vi "WIZARD.vi"() -> ()   [LabVIEW 2015]
uses:
  Controls/FGV_Options.ctl
  Controls/HID State.ctl
panel:
  out "String":string="System architecture (Windows Host and FPGA); LED Matrix (combination of 32x32 matrices in 2 rows and 3 columns); diving a little: row addressing are made in pair of n, n+15 rows. E.g., address 0 corresponds to rows 0 and 16 and ADRESS \"0xF\" or \"15\" corresponds to rows 15 and 31."
  in  "Button Back":bool
  out "2D Picture":picture
  out "Step Title":string
  out "Active Steps":string[](array[string])=["", "", "2. Coletando Dados Da Câmera!", "", "", "", ""]
  out "Steps Background":string[](array[string])=["Quer aprender como funciona a Demo?", "1. Vamos Começar", "2. Coletando Dados Da Câmera!", "3. Transformando em Vetor", "4. Enviando para o FPGA", "5. Colocando nas Memórias", "6. Gerando"]
  in  "Button Cancel":bool
  in  "Button Next":bool
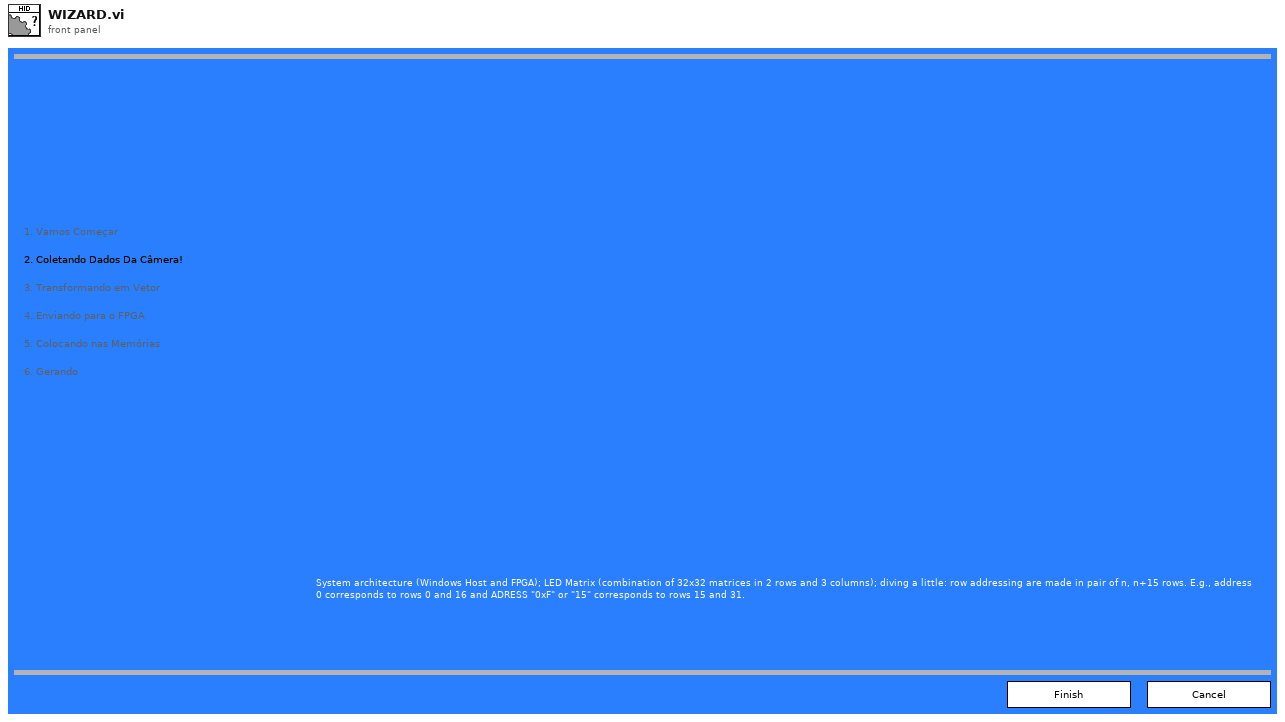
[diagram p1: front panel]
types:
  T1 = typedef "FGV_Options.ctl" = enum16{"Read from File", "Write to File", "Get", "Set"}
  T2 = cluster{"Steps":string[], "Images":picture[], "Step Counter":i32}
  T3 = typedef "HID Data.ctl" = cluster{"IMAQdx Session":T4, "Resampled Image":T5, "Low Level Grab":T5, "X Resolution":i32, "Y Resolution":i32, "Image Threshold":u8, "Reset Value":i32, "FIFO Timer":u16, "Row Timer":u32, "Memory Writer Timer":u8, "Color":enum16{"Green", "Blue", "Red", "White", "Pink", "Yellow", "Turquoise", "Black"}, "Top":bool[][], "Bottom":bool[][], "Timeout (ms)":i32, "Menu Tag":string, "Color Background":enum16{"Green", "Blue", "Red", "White", "Pink", "Yellow", "Turquoise", "Black"}, "FPGA VI Reference":refnum<k20>, "Next Steps":T6[], "Turn off LED Matrix":bool, "FPGA Alias":string, "FPGA Bitfile":path, "Localized Texts":cluster{"Status Text":cluster{"Status Text Table":string[], "Status Text Index":i32}, "Controls":cluster{"Control Text Table":string[], "Control Text Index":i32}, "Titles":cluster{"Titles Text Table":string[], "Titles Text Index":i32}}, "Language":u16}
  T4 = typedef "IMAQdx.ctl" = refnum<k21>
  T5 = typedef "IMAQ Image.ctl" = refnum<image>
  T6 = typedef "HID State.ctl" = enum16{"Initialize", "Set FPGA Parametes", "Set Camera Parameters", "Set LED Matrix Parameters", "Initialize FPGA Interface", "Initialize Camera", "Start FPGA VI", "Start Camera", "Wait for Event", "Update UI", "Acquire", "Process Image", "Get Boolean Arrays", "Send to FPGA", "Menu Pop-Up", "Menu Actions", "Handle Errors", "Close Camera", "Close FPGA", "Stop", "Exit"}
  T7 = enum8{"Enabled", "Disabled", "Disabled and Grayed Out"}
  T8 = typedef "imagedata.ctl" = cluster{"image type":i32, "image depth":i32, "image":u8[], "mask":u8[], "colors":u32[], "Rectangle":cluster{"left":i16, "top":i16, "right":i16, "bottom":i16}}
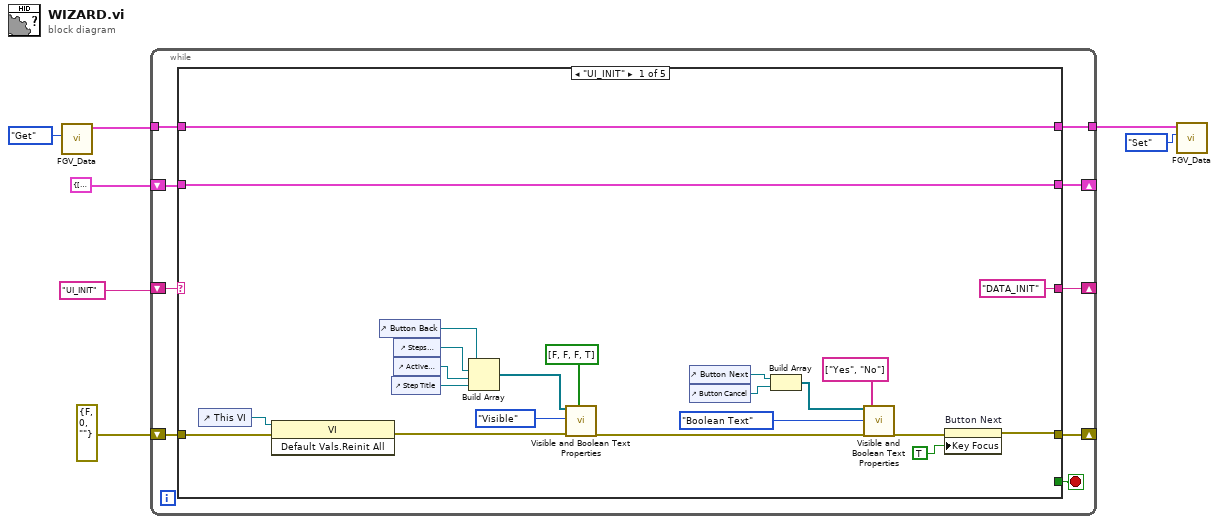
[diagram p0: block diagram]
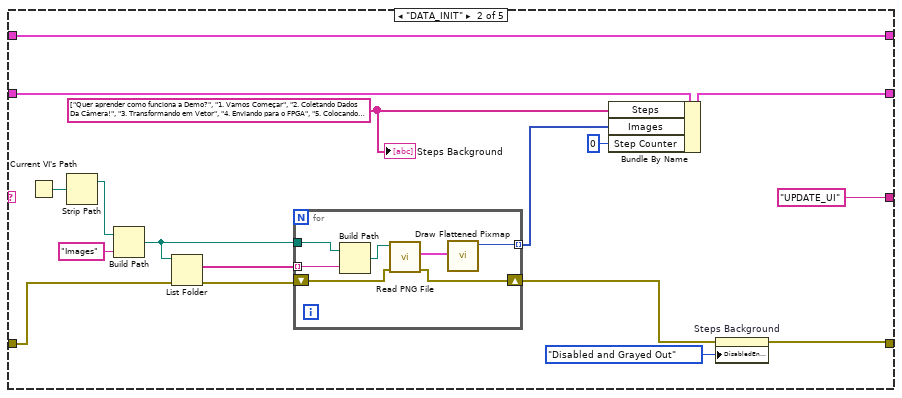
[diagram p2: hidden frame]
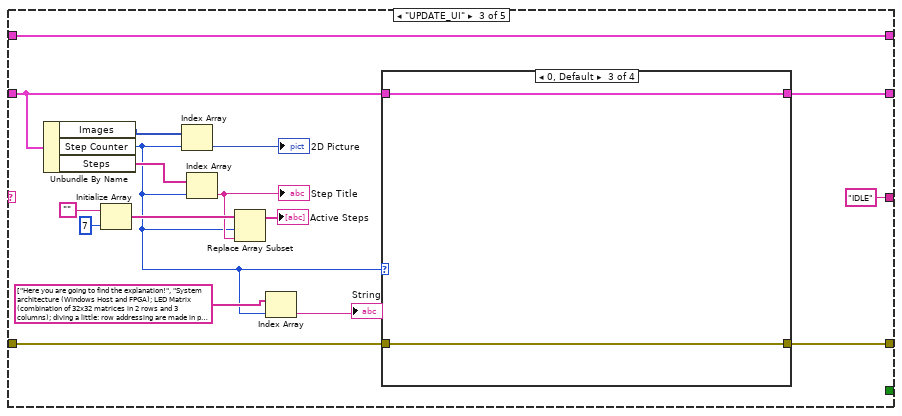
[diagram p3: hidden frame]
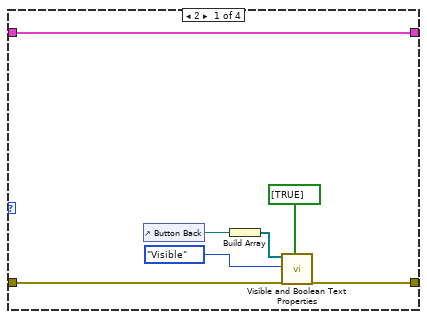
[diagram p4: hidden frame]
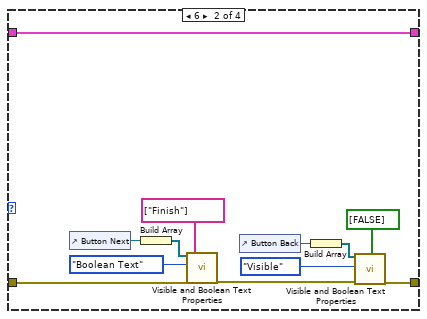
[diagram p5: hidden frame]
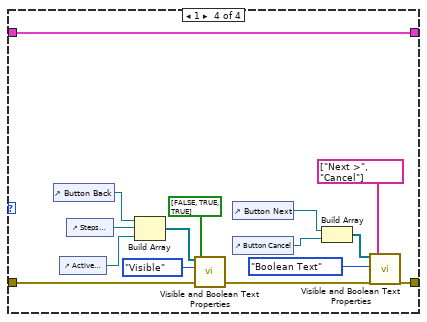
[diagram p6: hidden frame]
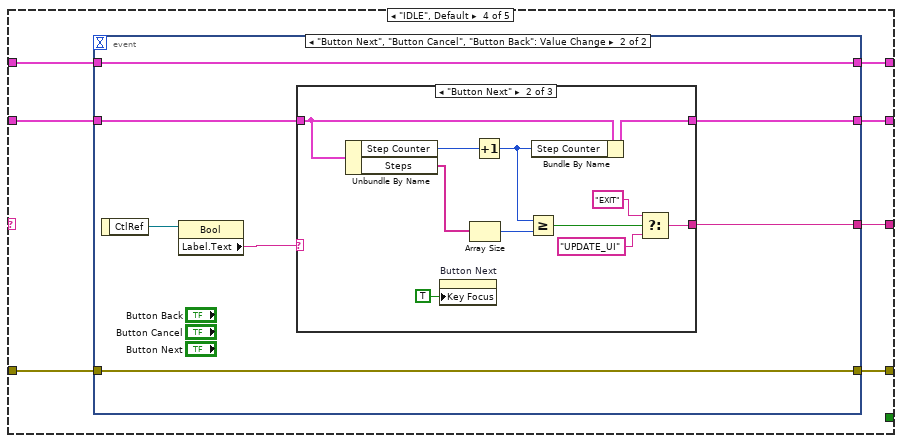
[diagram p7: hidden frame]
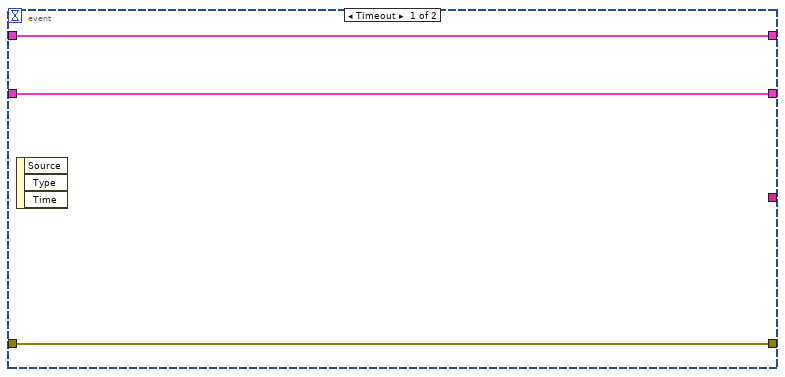
[diagram p8: hidden frame]
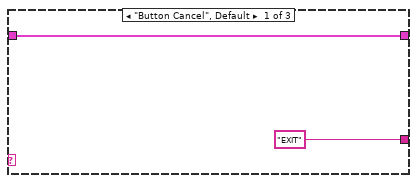
[diagram p9: hidden frame]
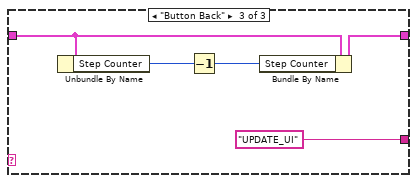
[diagram p10: hidden frame]
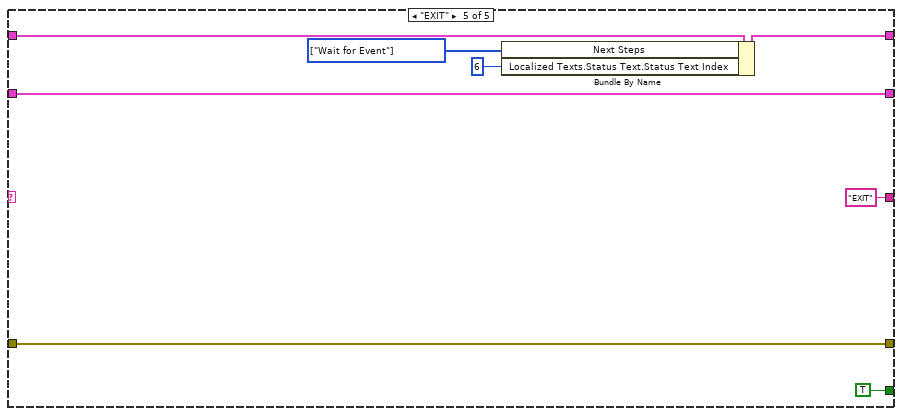
[diagram p11: hidden frame]
diagram:
  n1 = call "FGV_Data.vi"("Option"=FGV_Options."Get") -> ("Data Out"=w4:T3)  [unwired: 9 in, 1 out]
  n2 = while {
    shift-right: [w14] -> _
    shift-left: T2 {"Steps"=[], "Images"=[], "Step Counter"=0} -> [w15]
    shift-right: [w13] -> _
    shift-left: "UI_INIT" -> [w16]
    shift-right: [w11] -> _
    shift-left: errorcluster {"status"=FALSE, "code"=0, "source"=""} ("error constant") -> [w10]
    tunnel: w4 -> [w9]
    tunnel: [w8] -> w2
    stop <- w12 stop-if-true
    n3 = case shown="\"UI_INIT\"" w16 {
      tunnel: w15 -> [w38 w55 w71 w122 w158]
      tunnel: [w38 w53 w70 w121 w158] -> w14
      tunnel: ["DATA_INIT" "UPDATE_UI" "IDLE" w120 "EXIT"] -> w13
      tunnel: [_ _ _ _ TRUE] -> w12
      tunnel: [w19 w41 w68 w118 w155] -> w11
      tunnel: w10 -> [w18 w44 w69 w119 w155]
      tunnel: w9 -> [w17 w40 w66 w117 w154]
      tunnel: [w17 w40 w66 w116 w153] -> w8
      frame "UI_INIT" {
        n4 = control-ref of="This VI"() -> (w37:refnum<vi>)
        n5 = invoke class="VI" method="Default Vals.Reinit All"(reference=w37, error in=w18) -> (error out=w23:errorcluster)  [unwired: 1 in, 2 out]
        n6 = control-ref of="Button Back"() -> (w29:refnum<vi>)
        n7 = control-ref of="Step Title"() -> (w24:refnum<vi>)
        n8 = control-ref of="Steps Background"() -> (w25:refnum<vi>)
        n9 = control-ref of="Active Steps"() -> (w26:refnum<vi>)
        n10 = Build Array(w29, w25, w26, w24) -> (w27:refnum<vi>[])
        n11 = call "Visible and Boolean Text Properties.vi"("Control References"=w27, "Option"=enum16{"Visible", "Boolean Text"}."Visible", "error in (no error)"=w23, "Controls Visible Property Values"=bool[] [FALSE, FALSE, FALSE, TRUE]) -> ("error out"=w21:errorcluster)  [unwired: 15 in]
        n12 = control-ref of="Button Next"() -> (w31:refnum<vi>)
        n13 = control-ref of="Button Cancel"() -> (w32:refnum<vi>)
        n14 = Build Array(w31, w32) -> (w33:refnum<vi>[])
        n15 = call "Visible and Boolean Text Properties.vi"("Control References"=w33, "Option"=enum16{"Visible", "Boolean Text"}."Boolean Text", "error in (no error)"=w21, "Boolean Text Array"=string[] ["Yes", "No"]) -> ("error out"=w20:errorcluster)  [unwired: 15 in]
        n16 = property on="Button Next" class="Bool"(error in=w20, "Key Focus"=TRUE) -> (error out=w19:errorcluster)  [unwired: 1 in, 1 out]
      }
      frame "DATA_INIT" {
        w47 = string[] ["Quer aprender como funciona a Demo?", "1. Vamos Começar", "2. Coletando Dados Da Câmera!", "3. Transformando em Vetor", "4. Enviando para o FPGA", "5. Colocando nas Memórias", "6. Gerando"]
        n17 = Current VI's Path() -> (path=w52:path)
        n18 = Strip Path(path=w52) -> (stripped path=w39:path)  [unwired: 1 out]
        n19 = Build Path(base path=w39, name or relative path="Images") -> (appended path=w50:path)
        n20 = List Folder(path=w50, error in=w44) -> (filenames=w54:string[], error out=w43:errorcluster)  [unwired: 2 in, 2 out]
        n21 = for {
          tunnel: w54 -> [w62] mode=indexing
          tunnel: w50 -> [w61]
          tunnel: [w58] -> w49 mode=indexing
          shift-right: [w56] -> w42
          shift-left: w43 -> [w57]
          n22 = Build Path(base path=w61, name or relative path=w62) -> (appended path=w60:path)
          n23 = call <vilib>:"Read PNG File.vi"("error in (no error)"=w57, "path to PNG file"=w60) -> ("error out"=w56:errorcluster, "image data"=w59:T8)  [unwired: 7 in, 1 out]
          n24 = call <vilib>:"Draw Flattened Pixmap.vi"("image data"=w59) -> ("new picture"=w58:picture)  [unwired: 8 in]
        }
        n25 = Bundle By Name(cluster=w55, "Steps"=w47, "Images"=w49, "Step Counter"=0) -> (w53:T2)
        n26 = property on="Steps Background" class="Arr (strict)"(error in=w42, "DisabledEnum"=T7."Disabled and Grayed Out" ("Disabled")) -> (error out=w41:errorcluster)  [unwired: 1 in, 1 out]
        "Steps Background" <- w47
      }
      frame "UPDATE_UI" {
        n27 = Unbundle By Name(w71) -> ("Images"=w77:picture[], "Step Counter"=w63:i32, "Steps"=w67:string[])
        n28 = Initialize Array("", 7 ("dimension size")) -> (w75:string[])
        n29 = Index Array(array=w77, index=w63) -> (element=→"2D Picture":picture)
        n30 = Index Array(array=w67, index=w63) -> (element=w73:string)
        "Step Title" <- w73
        n31 = Replace Array Subset(array=w75, new element=w73, index=w63) -> (→"Active Steps":string[])
        n32 = Index Array(array=string[] ["Here you are going to find the explanation!", "System architecture (Windows Host and FPGA); LED Matrix (combination of 32x32 matrices in 2 rows and 3 columns); diving a little: row addressing are made in pair of n, n+15 rows. E.g., address 0 corresponds to rows 0 and 16 and ADRESS \"0xF\" or \"15\" corresponds to rows 15 and 31.", "Camera acquires image", "Image is processed. The image is casted into a 8-bit Grayscale image and then resampled to become a 96x64 pixels image. Can you guess why this is made? Ans. To match the number of pixels in the LED Matrix.", "Image is converted into a 2D boolean array. This array is divided in two blocks.", "Host sends n concatenated to n+15 1D array ( column values for a row) to FPGA via DMA FIFO.", "Down in FPGA each \"n concatenated to n+15\" row is split in two separated \"n\" and \"n+15\" 1D arrays. ", "FPGA sets the address for each row and then the n and n+15 are indexed so that each column value is passed to FPGA digital Outputs. Before writing out each column pixel, FPGA determines if this pixel will contain the foreground or background color."], index=w63) -> (element=→"String":string)
        n33 = case shown="0, Default" w63 {
          tunnel: w71 -> [w86 w98 w100 w115]
          tunnel: [w86 w98 w100 w115] -> w70
          tunnel: w69 -> [w81 w88 w99 w102]
          tunnel: [w80 w89 w99 w103] -> w68
          frame 2 {
            n34 = control-ref of="Button Back"() -> (w84:refnum<vi>)
            n35 = Build Array(w84) -> (w83:refnum<vi>[])
            n36 = call "Visible and Boolean Text Properties.vi"("Control References"=w83, "Option"=enum16{"Visible", "Boolean Text"}."Visible", "error in (no error)"=w81, "Controls Visible Property Values"=bool[] [TRUE]) -> ("error out"=w80:errorcluster)  [unwired: 15 in]
          }
          frame 6 {
            n37 = control-ref of="Button Next"() -> (w93:refnum<vi>)
            n38 = Build Array(w93) -> (w94:refnum<vi>[])
            n39 = call "Visible and Boolean Text Properties.vi"("Control References"=w94, "Option"=enum16{"Visible", "Boolean Text"}."Boolean Text", "error in (no error)"=w88, "Boolean Text Array"=string[] ["Finish"]) -> ("error out"=w87:errorcluster)  [unwired: 15 in]
            n40 = control-ref of="Button Back"() -> (w96:refnum<vi>)
            n41 = Build Array(w96) -> (w95:refnum<vi>[])
            n42 = call "Visible and Boolean Text Properties.vi"("Control References"=w95, "Option"=enum16{"Visible", "Boolean Text"}."Visible", "error in (no error)"=w87, "Controls Visible Property Values"=bool[] [FALSE]) -> ("error out"=w89:errorcluster)  [unwired: 15 in]
          }
          frame 0, Default {
          }
          frame 1 {
            n43 = control-ref of="Button Back"() -> (w109:refnum<vi>)
            n44 = control-ref of="Active Steps"() -> (w105:refnum<vi>)
            n45 = control-ref of="Steps Background"() -> (w104:refnum<vi>)
            n46 = Build Array(w109, w104, w105) -> (w106:refnum<vi>[])
            n47 = call "Visible and Boolean Text Properties.vi"("Control References"=w106, "Option"=enum16{"Visible", "Boolean Text"}."Visible", "error in (no error)"=w102, "Controls Visible Property Values"=bool[] [FALSE, TRUE, TRUE]) -> ("error out"=w101:errorcluster)  [unwired: 15 in]
            n48 = control-ref of="Button Next"() -> (w111:refnum<vi>)
            n49 = control-ref of="Button Cancel"() -> (w112:refnum<vi>)
            n50 = Build Array(w111, w112) -> (w113:refnum<vi>[])
            n51 = call "Visible and Boolean Text Properties.vi"("Control References"=w113, "Option"=enum16{"Visible", "Boolean Text"}."Boolean Text", "error in (no error)"=w101, "Boolean Text Array"=string[] ["Next >", "Cancel"]) -> ("error out"=w103:errorcluster)  [unwired: 15 in]
          }
        }
      }
      frame "IDLE", Default {
        n52 = event shown="[1] \"Button Next\", \"Button Cancel\", \"Button Back\": Value Change" {
          selector: _ -> [_ _]
          dyn-events: _ -> [_ _]
          timeout: _ -> [_ _]
          tunnel: w122 -> [w125 w128]
          tunnel: [w125 w130] -> w121
          tunnel: [_ w129] -> w120
          tunnel: w119 -> [w124 w127]
          tunnel: [w124 w127] -> w118
          tunnel: w117 -> [w123 w126]
          tunnel: [w123 w126] -> w116
          event Timeout {
            n53 = event-data() -> ()  [unwired: 1 in, 3 out]
          }
          event "Button Next", "Button Cancel", "Button Back": Value Change {
            n54 = event-data() -> ("CtlRef"=w132:refnum<vi>)  [unwired: 1 in]
            n55 = property class="Bool"(reference=w132) -> ("Label.Text"=w131:string)  [unwired: 1 in, 2 out]
            n56 = case shown="\"Button Next\"" w131 {
              tunnel: w128 -> [w134 w144 w149]
              tunnel: [w134 w145 w150] -> w130
              tunnel: ["EXIT" w136 "UPDATE_UI"] -> w129
              frame "Button Cancel", Default {
              }
              frame "Button Next" {
                n57 = Unbundle By Name(w144) -> ("Step Counter"=w143:i32, "Steps"=w141:string[])
                n58 = property on="Button Next" class="Bool"("Key Focus"=TRUE) -> ()  [unwired: 2 in, 2 out]
                n59 = Array Size(array=w141) -> (size(s)=w142:i32)
                n60 = Increment(x=w143) -> (x+1=w140:i32)
                n61 = Greater Or Equal?(x=w140, y=w142) -> (x >= y?=w137:bool)
                n62 = Bundle By Name(cluster=w144, "Step Counter"=w140) -> (w145:T2)
                n63 = Select(t="EXIT", s=w137, f="UPDATE_UI") -> (s? t:f=w136:string)
              }
              frame "Button Back" {
                n64 = Unbundle By Name(w149) -> ("Step Counter"=w148:i32)
                n65 = Decrement(x=w148) -> (x-1=w147:i32)
                n66 = Bundle By Name(cluster=w149, "Step Counter"=w147) -> (w150:T2)
              }
            }
          }
        }
      }
      frame "EXIT" {
        w152 = T6[] [enum."Wait for Event"] items=["Initialize", "Set FPGA Parametes", "Set Camera Parameters", "Set LED Matrix Parameters", "Initialize FPGA Interface", "Initialize Camera", "Start FPGA VI", "Start Camera", "Wait for Event", "Update UI", "Acquire", "Process Image", "Get Boolean Arrays", "Send to FPGA", "Menu Pop-Up", "Menu Actions", "Handle Errors", "Close Camera", "Close FPGA", "Stop", "Exit"] ("Array")
        n67 = Bundle By Name(cluster=w154, "Next Steps"=w152, "Localized Texts.Status Text.Status Text Index"=6 ("Status")) -> (w153:T3)
      }
    }
  }
  n68 = call "FGV_Data.vi"("Option"=FGV_Options."Set", "Data In"=w2) -> ()  [unwired: 8 in, 2 out]
